vi "Stop Core.vi"(10 "final error code":i32, 11 "Actor in":refnum<class "Actor1_BasicNoLib_N_4.0.0.lvclass">) -> (3 "Actor out":refnum<class "Actor1_BasicNoLib_N_4.0.0.lvclass">)   [LabVIEW 2014, in "Actor1_BasicNoLib_N_4.0.0.lvclass"]
uses:
  <resource>/Framework/Providers/Open_GDS/ClassProviders/ActorFramework/4.0.0/Actor1_BasicNoLib_N_4.0.0/Actor1_BasicNoLib_N_4.0.0_class/Actor1_BasicNoLib_N_4.0.0.lvclass
  <vilib>/ActorFramework/Actor/Actor.lvclass
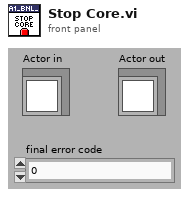
[diagram p1: front panel]
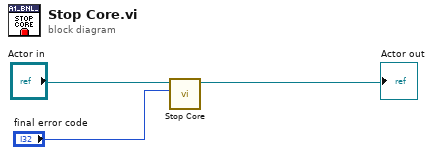
[diagram p0: block diagram]
diagram:
  n1 = call-parent "Stop Core.vi"("final error code"="final error code", "Actor in"="Actor in") -> ("Actor out"=→"Actor out":refnum<class "Actor1_BasicNoLib_N_4.0.0.lvclass">)  [unwired: 9 in]
